vi "cal2kim18.vi"(11 "6DOF Calibration":T2) -> (3 "Kim18 calibration":T1)   [LabVIEW 2024]
uses:
  kim18_calibration.ctl
  6dof_calibration.ctl
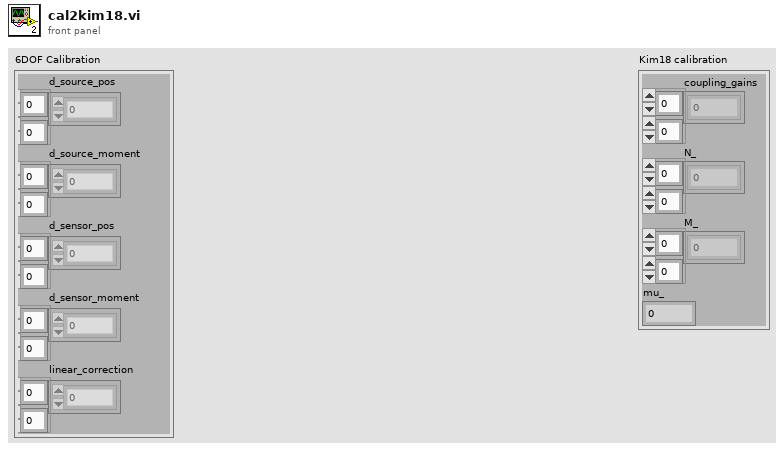
[diagram p1: front panel]
types:
  T1 = typedef "kim18_calibration.ctl" = cluster{"coupling_gains":dbl[][], "N_":dbl[][], "M_":dbl[][], "mu_":dbl}
  T2 = typedef "6dof_calibration.ctl" = cluster{"d_source_pos":dbl[][], "d_source_moment":dbl[][], "d_sensor_pos":dbl[][], "d_sensor_moment":dbl[][], "linear_correction":dbl[][]}
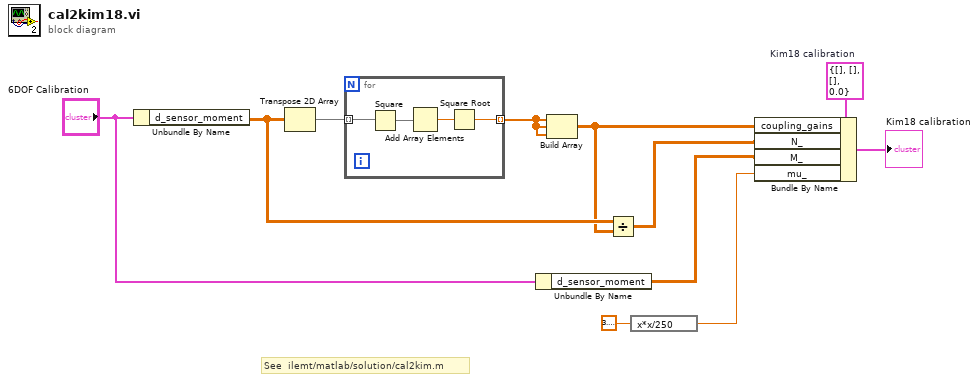
[diagram p0: block diagram]
diagram:
  w9 = T1 {"coupling_gains"=[], "N_"=[], "M_"=[], "mu_"=0.0}  # Kim18 calibration
  # "See  ilemt/matlab/solution/cal2kim.m"
  n1 = Unbundle By Name("6DOF Calibration") -> ("d_sensor_moment"=w8:dbl[][])
  n2 = Transpose 2D Array(2D array=w8) -> (transposed array=w11:dbl[][])
  n3 = for {
    tunnel: w11 -> [w15] mode=indexing
    tunnel: [w12] -> w10 mode=indexing
    n4 = Square(x=w15) -> (x^2=w14:dbl[])
    n5 = Add Array Elements(numeric array=w14) -> (sum=w13:dbl)
    n6 = Square Root(x=w13) -> (sqrt(x)=w12:dbl)
  }
  n7 = Unbundle By Name("6DOF Calibration") -> ("d_sensor_moment"=w4:dbl[][])
  n8 = Build Array(w10, w10, w10) -> (w7:dbl[][])
  n9 = Divide(x=w8, y=w7) -> (x/y=w6:dbl[][])
  n10 = expression code="x*x/250"(3.141592653589793) -> (w2:dbl)
  n11 = Bundle By Name(cluster=w9, "coupling_gains"=w7, "N_"=w6, "M_"=w4, "mu_"=w2) -> (→"Kim18 calibration":T1)
